vi "Data process.vi"(8 "error in":errorcluster caption="错误输入", 10 "Data Read":string, 11 "CMD":string) -> (0 "error IO":errorcluster, 3 "Data_Float":dbl)   [LabVIEW 2015]
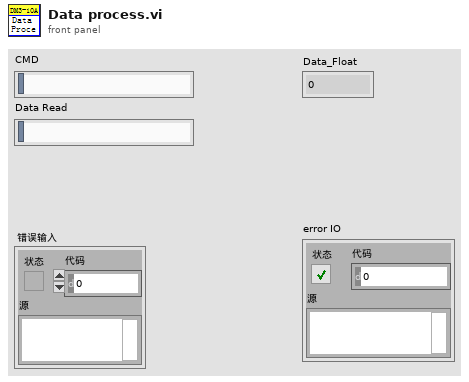
[diagram p1: front panel]
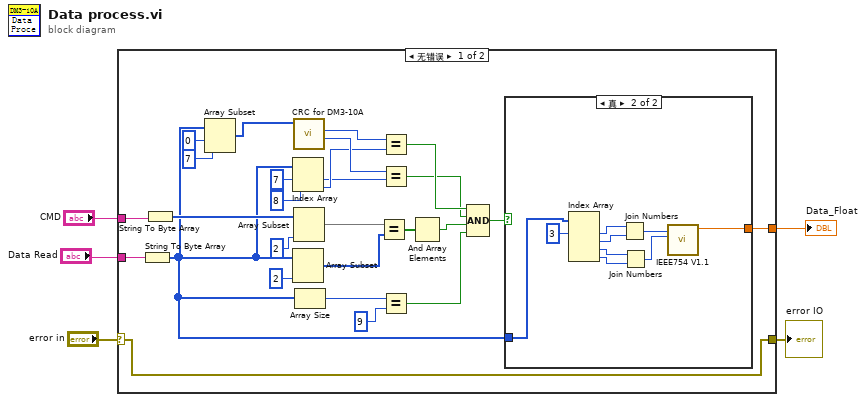
[diagram p0: block diagram]
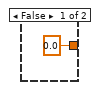
[diagram p2: hidden frame]
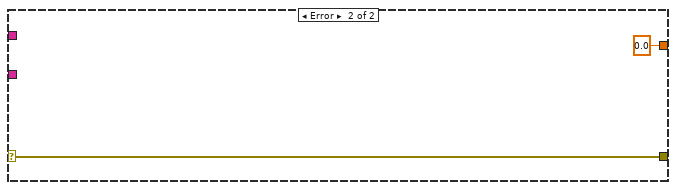
[diagram p3: hidden frame]
diagram:
  n1 = case shown="无错误" "error in" {
    selector: "error in" -> [w10 w43]
    tunnel: "Data Read" -> [w32 _]
    tunnel: "CMD" -> [w31 _]
    tunnel: [w11 0.0 ("输出浮点型")] -> w2
    tunnel: [w10 w43] -> w1
    frame No Error {
      n2 = String To Byte Array(string=w32) -> (unsigned byte array=w9:u8[])
      n3 = String To Byte Array(string=w31) -> (unsigned byte array=w26:u8[])
      n4 = Array Subset(array=w9, index=0 ("索引"), length=7 ("长度")) -> (w8:u8[])
      n5 = Index Array(array=w9, index #1=7 ("索引"), index #2=8 ("索引")) -> (element #1=w20:u8, element #2=w21:u8)
      n6 = Array Subset(array=w9, length=2 ("长度")) -> (w27:u8[])  [unwired: 1 in]
      n7 = call "CRC for DM3-10A.vi"("CMD"=w8) -> ("CRCLo"=w22:u8, "CRCHi"=w23:u8)  [unwired: 8 in, 1 out]
      n8 = Array Subset(array=w26, length=2 ("长度")) -> (w28:u8[])  [unwired: 1 in]
      n9 = Array Size(array=w9) -> (size(s)=w19:i32)
      n10 = Equal?(x=w28, y=w27) -> (x = y?=w14:bool[])
      n11 = Equal?(x=w23, y=w21) -> (x = y?=w17:bool)
      n12 = Equal?(x=w22, y=w20) -> (x = y?=w16:bool)
      n13 = Equal?(x=w19, y=9) -> (x = y?=w15:bool)
      n14 = And Array Elements(Boolean array=w14) -> (logical AND=w13:bool)
      n15 = Compound Arithmetic op=AND ("复合运算")(w17, w16, w13, w15) -> (w12:bool)
      n16 = case shown="真" w12 {
        tunnel: w9 -> [_ w36]
        tunnel: [0.0 ("输出浮点型") w35] -> w11
        frame False {
        }
        frame True {
          n17 = Index Array(array=w36, index #1=3 ("索引")) -> (element #1=w40:u8, element #2=w41:u8, element #3=w42:u8, element #4=w34:u8)  [unwired: 3 in]
          n18 = Join Numbers(hi=w40, lo=w41) -> ((hi.lo)=w37:u16)
          n19 = Join Numbers(hi=w42, lo=w34) -> ((hi.lo)=w38:u16)
          n20 = call "IEEE754 V1.1.vi"("低位16"=w38, "高位16"=w37) -> ("输出浮点型"=w35:dbl)  [unwired: 8 in, 1 out]
        }
      }
    }
    frame Error {
    }
  }
  "Data_Float" <- w2
  "error IO" <- w1
